vi "DAQ 디지털 버튼 입출력 실습.vi"() -> ()   [LabVIEW 2020]
uses:
  <vilib>/DAQmx/read.llb/DAQmx Read (Digital 1D Bool 1Chan 1Samp).vi
  <vilib>/DAQmx/write.llb/DAQmx Write (Digital 1D Bool 1Chan 1Samp).vi
  <vilib>/DAQmx/create/channels.llb/DAQmx Create Channel (DI-Digital Input).vi
  <vilib>/DAQmx/create/channels.llb/DAQmx Create Channel (DO-Digital Output).vi
  <vilib>/DAQmx/miscellaneous.llb/DAQmx Fill In Error Info.vi
panel:
  out "data":bool[](array[boolean]) caption="데이터"
  in  "정지":bool
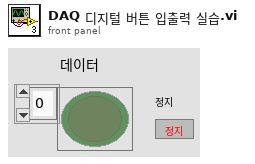
[diagram p1: front panel]
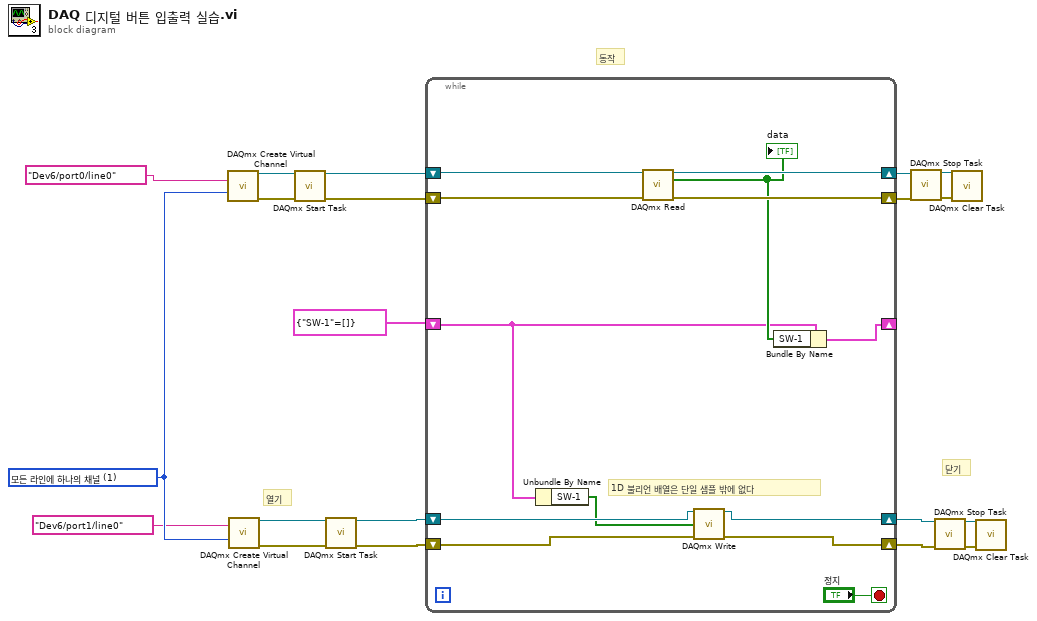
[diagram p0: block diagram]
diagram:
  w13 = 1 items=["각 라인에 하나의 채널", "모든 라인에 하나의 채널"] ("line grouping")
  # "열기"
  # "닫기"
  # "동작"
  n1 = call-poly <vilib>:"DAQmx Create Virtual Channel.vi"("lines"=tag "Dev6/port0/line0", "line grouping"=w13) -> ("task out"=w15:refnum<k21>, "error out"=w14:errorcluster)  [unwired: 12 in]
  n2 = call-poly <vilib>:"DAQmx Create Virtual Channel.vi"("lines"=tag "Dev6/port1/line0", "line grouping"=w13) -> ("task out"=w5:refnum<k21>, "error out"=w4:errorcluster)  [unwired: 12 in]
  n3 = call <vilib>:"DAQmx Start Task.vi"("task/channels in"=w15, "error in"=w14) -> ("task out"=w12:refnum<k21>, "error out"=w11:errorcluster)  [unwired: 12 in]
  n4 = call <vilib>:"DAQmx Start Task.vi"("task/channels in"=w5, "error in"=w4) -> ("task out"=w20:refnum<k21>, "error out"=w19:errorcluster)  [unwired: 12 in]
  n5 = while {
    shift-right: [w31] -> w18
    shift-left: w20 -> [w33]
    shift-right: [w30] -> w17
    shift-left: w19 -> [w32]
    shift-right: [w26] -> w8
    shift-left: w12 -> [w29]
    shift-right: [w27] -> w7
    shift-left: w11 -> [w28]
    shift-right: [w23] -> _
    shift-left: cluster{"SW-1":bool[]} {"SW-1"=[]} -> [w22]
    stop <- "정지" stop-if-true
    # "1D 불리언 배열은 단일 샘플 밖에 없다"
    n6 = Unbundle By Name(w22) -> ("SW-1"=w21:bool[])
    n7 = call-poly <vilib>:"DAQmx Read.vi"("task/channels in"=w29, "error in"=w28) -> ("task out"=w26:refnum<k21>, "data"=w24:bool[], "error out"=w27:errorcluster)  [unwired: 11 in]
    "data" <- w24
    n8 = call-poly <vilib>:"DAQmx Write.vi"("task/channels in"=w33, "data"=w21, "error in"=w32) -> ("task out"=w31:refnum<k21>, "error out"=w30:errorcluster)  [unwired: 10 in, 1 out]
    n9 = Bundle By Name(cluster=w22, "SW-1"=w24) -> (w23:cluster{"SW-1":bool[]})
  }
  n10 = call <vilib>:"DAQmx Stop Task.vi"("task/channels in"=w8, "error in"=w7) -> ("task out"=w9:refnum<k21>, "error out"=w10:errorcluster)  [unwired: 12 in]
  n11 = call <vilib>:"DAQmx Stop Task.vi"("task/channels in"=w18, "error in"=w17) -> ("task out"=w3:refnum<k21>, "error out"=w2:errorcluster)  [unwired: 12 in]
  n12 = call <vilib>:"DAQmx Clear Task.vi"("task in"=w9, "error in"=w10) -> ()  [unwired: 13 in, 1 out]
  n13 = call <vilib>:"DAQmx Clear Task.vi"("task in"=w3, "error in"=w2) -> ()  [unwired: 13 in, 1 out]
